vi "Teleop.vi"(10 "Match Info":T1={"Autonomous Elapsed Seconds"=0.0, "TeleOp Elapsed Seconds"=0.0, "Disabled Elapsed Seconds"=0.0, "Visited Autonomous"=FALSE, "Visited TeleOp"=FALSE, "Visited Disabled"=FALSE, "Autonomous Settings"={"Autonomous Style"=enum."Independent", "VI Refnum"=refnum}}, 11 "Call Context":T2) -> ()   [LabVIEW 2015]
doc: "This VI is called for each TeleOp packet received from the DS where the robot is not disabled. It is often used to read from the joysticks and update I/O or to update setpoints for timed control loops. It should complete and return within 20 milliseconds or it may miss DS packets."
uses:
  <vilib>/Rock Robotics/WPI/DriverStation/WPI_DriverStationDerivedRobotMode.ctl
  <vilib>/Rock Robotics/WPI/DriverStation/WPI_DriverStationMatch Info.ctl
  <vilib>/Rock Robotics/Network Tables/NT Read Boolean.vi
  <vilib>/Rock Robotics/Network Tables/NT Read Number.vi
  <vilib>/Rock Robotics/WPI/Utilities/WPI_GetSetVariantRefNum.vi
  Robot Global Data.vi
  <vilib>/Rock Robotics/Network Tables/NT Write Numeric Array.vi
  <vilib>/Rock Robotics/Network Tables/NT Write Boolean Array.vi
panel:
  in  "Fire":bool
  in  "Ball Intake":bool
  in  "Drive Mode":enum16{"Tank Drive", "Arcade Drive"}(ring)
  in  "Controller Mode":enum16{"X-Box Controller", "Joysticks"}(ring)
  out "Sample Slider 0":dbl(slide) scale=0.0..5.0
  out "Sample Boolean 1":bool
  out "Sample Boolean 0":bool
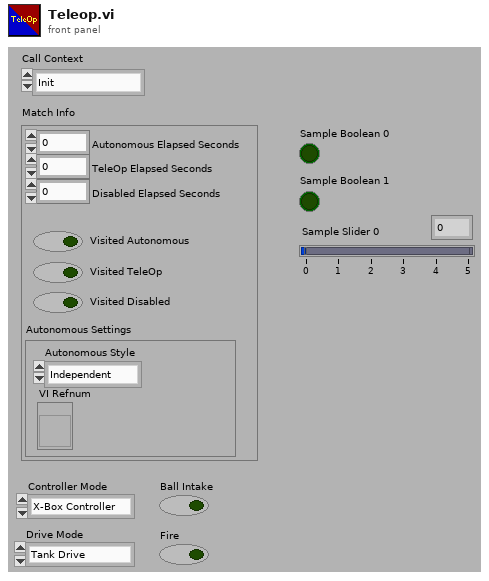
[diagram p1: front panel]
types:
  T1 = typedef "WPI_DriverStationMatch Info.ctl" = cluster{"Autonomous Elapsed Seconds":dbl, "TeleOp Elapsed Seconds":dbl, "Disabled Elapsed Seconds":dbl, "Visited Autonomous":bool, "Visited TeleOp":bool, "Visited Disabled":bool, "Autonomous Settings":cluster{"Autonomous Style":enum16{"Iterative", "Independent"}, "VI Refnum":refnum<vi>}}
  T2 = typedef "WPI_DriverStationDerivedRobotMode.ctl" = enum16{"Init", "Execute", "Stop"}
  T3 = typedef "WPI_RobotDriveDevRef.ctl" = cluster{"DevStatus":errorcluster, "Motors[]":T4[], "Square Inputs":bool, "Max Output":dbl}
  T4 = typedef "WPI_MotorControlDeviceRef.ctl" = cluster{"DeviceStatus":errorcluster, "Type":T5, "PWM":cluster{"PWM Channel":T6, "DeadBand":T7}, "CAN":cluster{"Device Number":u8, "Control Mode":T8, "Semaphore":T9, "Max Vout":dbl, "TalonSRX Control Mode":T10}, "Invert":bool}
  T5 = typedef "WPI_MotorControlType.ctl" = enum16{"PWM", "CAN", "CANTalonSRX"}
  T6 = typedef "FPGA_DIOPWMChannel.ctl" = enum8{"PWM 0", "PWM 1", "PWM 2", "PWM 3", "PWM 4", "PWM 5", "PWM 6", "PWM 7", "PWM 8", "PWM 9", "PWM MXP 0", "PWM MXP 1", "PWM MXP 2", "PWM MXP 3", "PWM MXP 4", "PWM MXP 5", "PWM MXP 6", "PWM MXP 7", "PWM MXP 8", "PWM MXP 9", "Invalid"}
  T7 = typedef "WPI_PWMDeadband.ctl" = cluster{"Name":string, "maxPositivePwm":i32, "minPositivePwm":i32, "centerPwm":i32, "maxNegativePwm":i32, "minNegativePwm":i32, "angularRange":u16}
  T8 = typedef "WPI_CANJaguar_ControlMode.ctl" = enum8{"Percent VBus", "Current", "Speed", "Position", "Voltage"}
  T9 = typedef "Semaphore RefNum" = refnum<k1>
  T10 = typedef "WPI_CANTalonSRX_APIControlMode.ctl" = enum8{"Percent VBus", "Speed", "Position", "Slave", "Unchanged / Invalid", "Voltage Compensation", "Current", "Motion Profile"}
  T11 = typedef "WPI_JoystickDevRef.ctl" = cluster{"Device":T12}
  T12 = typedef "WPI_JoystickDeviceEnum.ctl" = enum16{"USB 0", "USB 1", "USB 2", "USB 3", "USB 4", "USB 5"}
  T13 = cluster{"Ball Shooter Operation":enum16{"Ball Intake", "Fire Ball Shooter", "Aim Ball Shooter"}}
  T14 = enum16{"Ball Intake", "Fire Ball Shooter", "Aim Ball Shooter"}
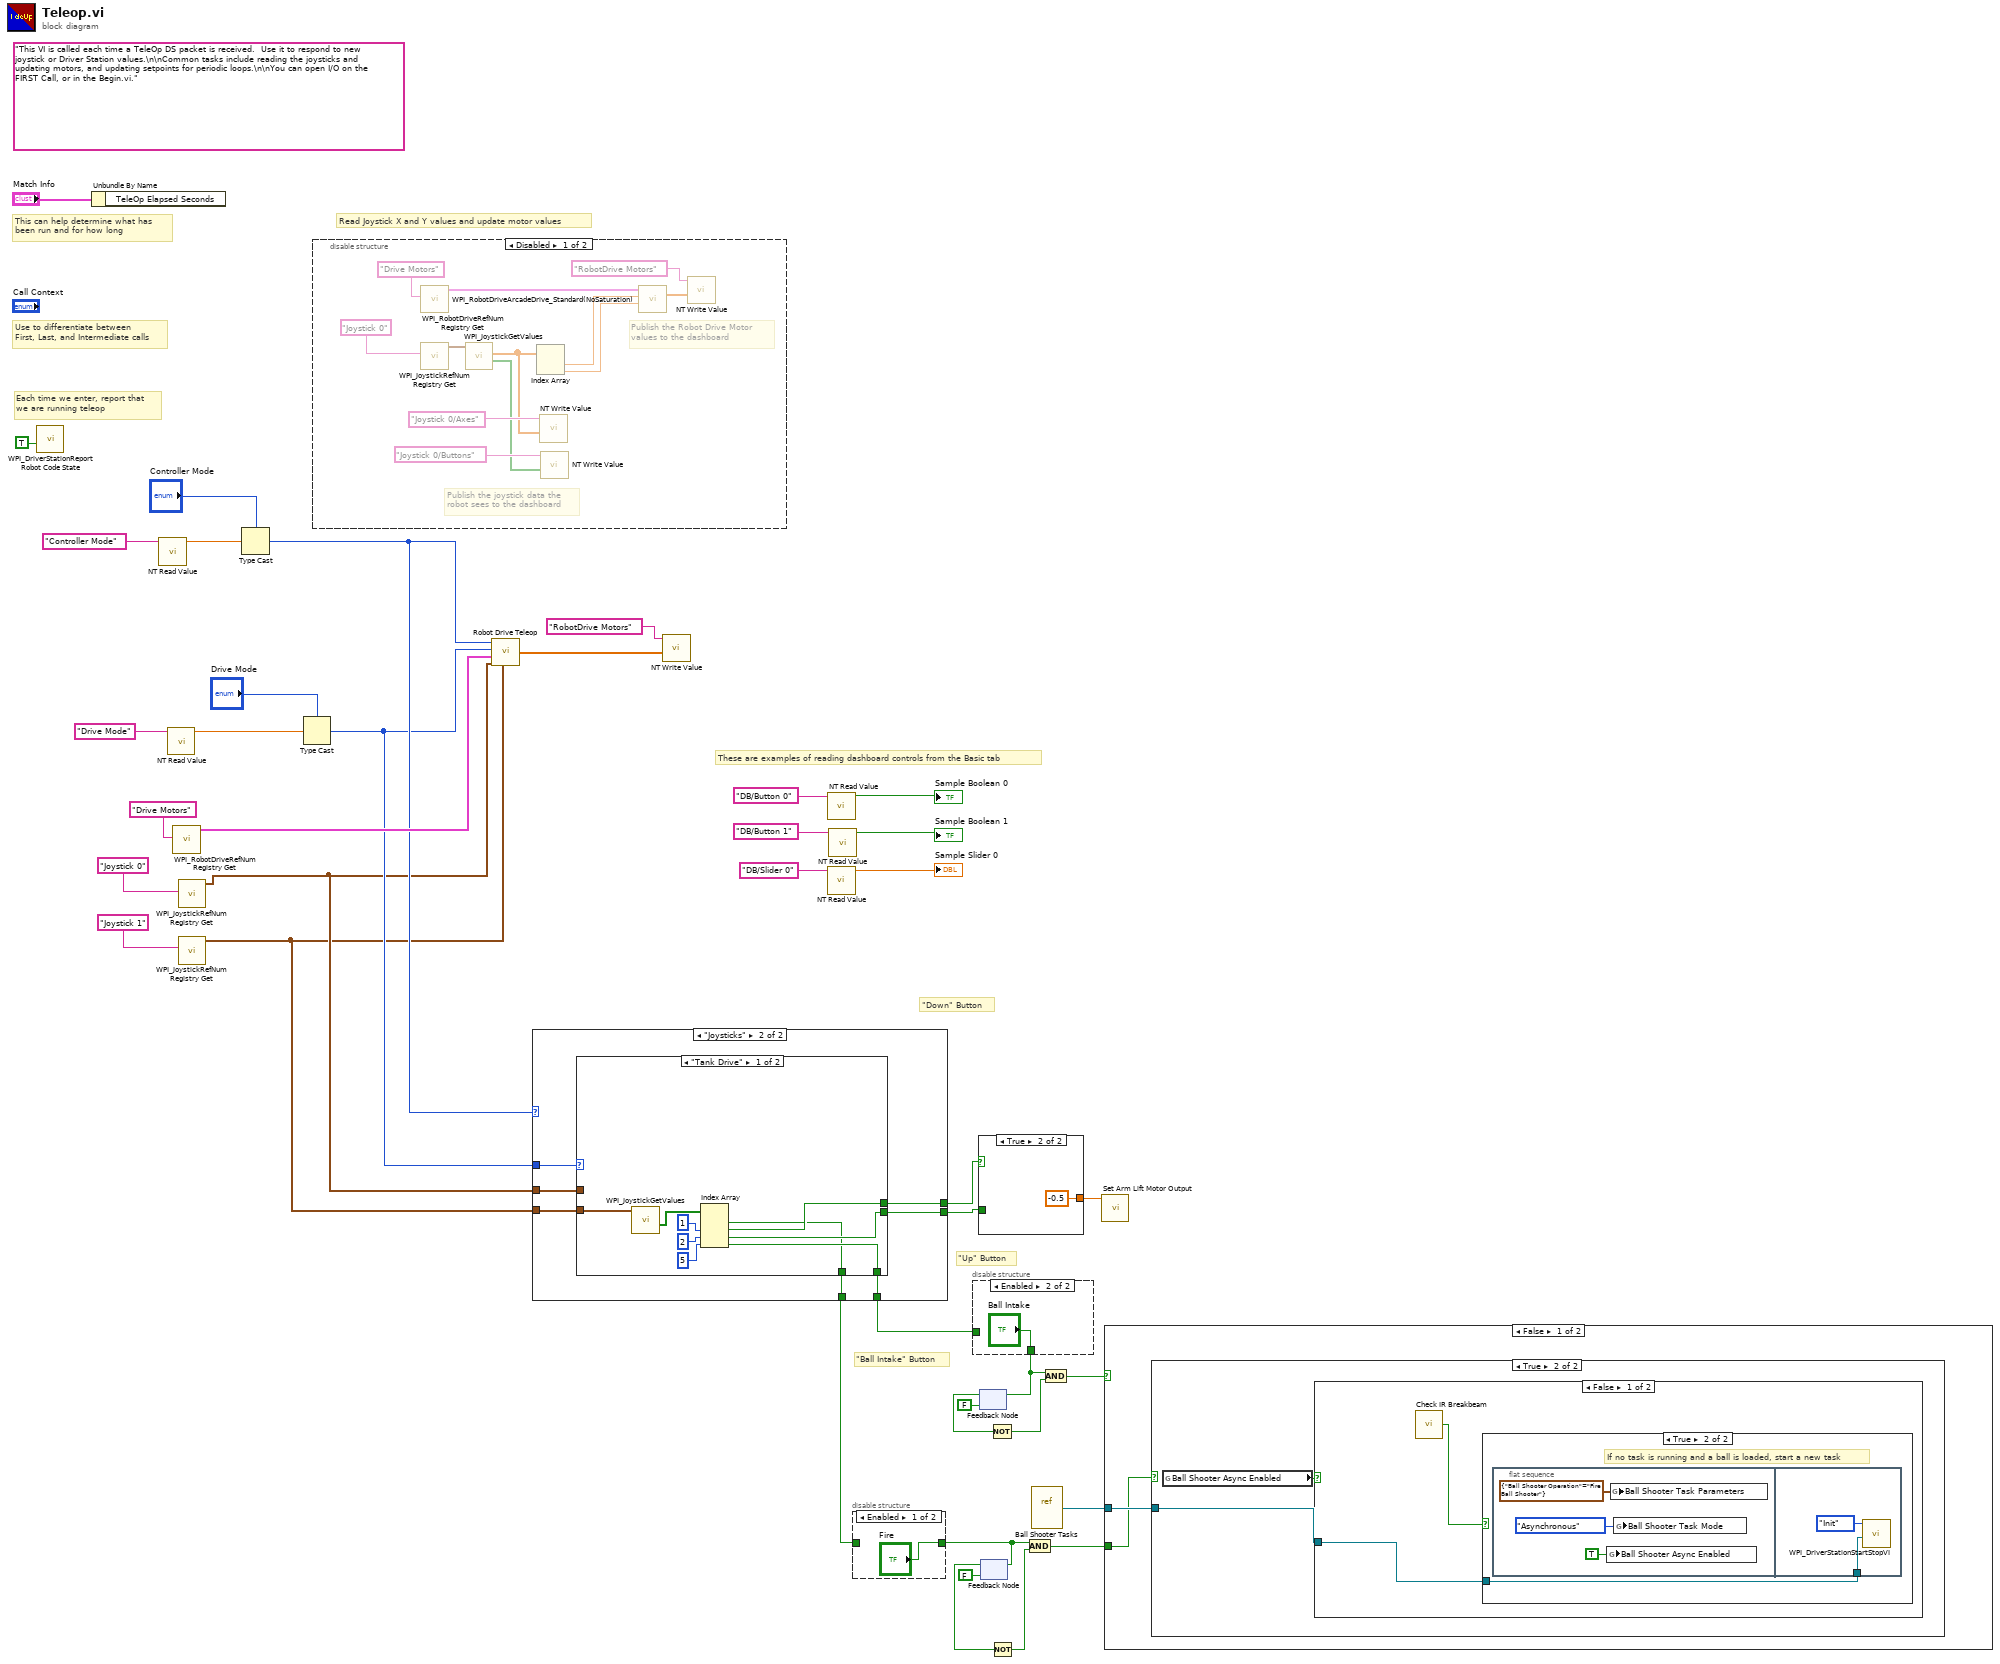
[diagram p0: block diagram]
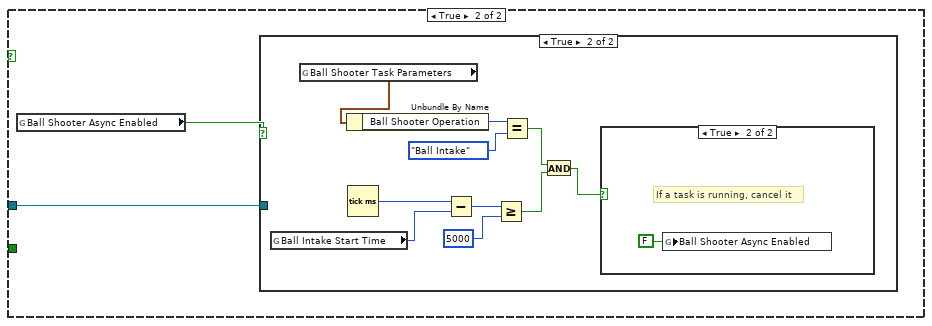
[diagram p7: hidden frame]
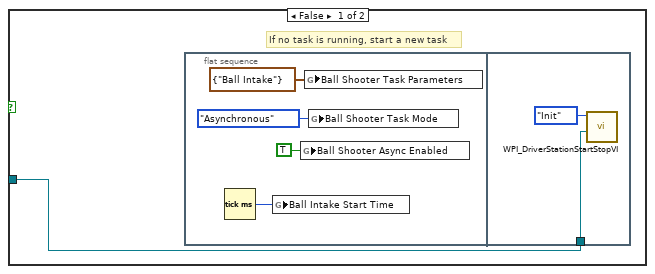
[diagram p8: hidden frame]
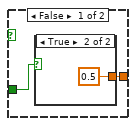
[diagram p10: hidden frame]
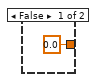
[diagram p11: hidden frame]
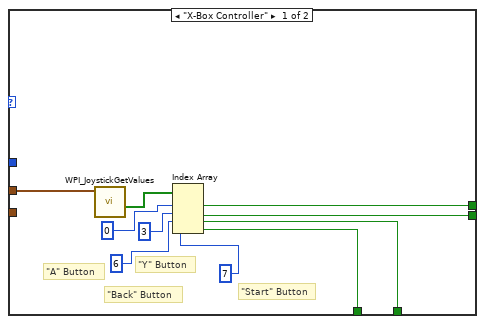
[diagram p12: hidden frame]
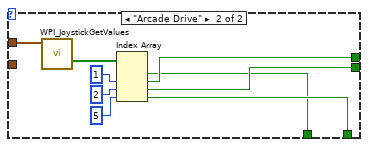
[diagram p13: hidden frame]
diagram:
  (unwired) "This VI is called each time a TeleOp DS packet is received.  Use it to respond to new joystick or Driver Station values.\n\nCommon tasks include reading the joysticks and updating motors, and updating setpoints for periodic loops.\n\nYou can open I/O on the FIRST Call, or in the Begin.vi."
  # "\"Ball Intake\" Button"
  # "\"Up\" Button"
  # "\"Down\" Button"
  # "These are examples of reading dashboard controls from the Basic tab"
  # "Each time we enter, report that\nwe are running teleop"
  # "Use to differentiate between\nFirst, Last, and Intermediate calls"
  # "This can help determine what has\nbeen run and for how long"
  # "Read Joystick X and Y values and update motor values"
  n1 = call <vilib>:"WPI_DriverStationReport Robot Code State.vi"("TeleOp"=TRUE ("Autonomous")) -> ()  [unwired: 10 in, 1 out]
  n2 = Unbundle By Name("Match Info") -> ()  [unwired: 1 out]
  n3 = call-poly <vilib>:"NT Read Value.vi"("Name"="Controller Mode") -> ("Numeric"=w31:dbl)  [unwired: 9 in, 1 out]
  n4 = call-poly <vilib>:"NT Read Value.vi"("Name"="Drive Mode") -> ("Numeric"=w27:dbl)  [unwired: 9 in, 1 out]
  n5 = call <vilib>:"WPI_RobotDriveRefNum Registry Get.vi"("refnum name"="Drive Motors") -> ("RobotDriveDevRef"=w25:T3)  [unwired: 1 in, 9 out]
  n6 = call <vilib>:"WPI_JoystickRefNum Registry Get.vi"("refnum name"="Joystick 0") -> ("JoystickDevRef"=w18:T11)  [unwired: 1 in, 9 out]
  n7 = call <vilib>:"WPI_JoystickRefNum Registry Get.vi"("refnum name"="Joystick 1") -> ("JoystickDevRef"=w17:T11)  [unwired: 1 in, 9 out]
  n8 = Type Cast(type="Controller Mode", x=w31) -> (*(type *) &x=w20:enum16{"X-Box Controller", "Joysticks"})
  n9 = Type Cast(type="Drive Mode", x=w27) -> (*(type *) &x=w19:enum16{"Tank Drive", "Arcade Drive"})
  n10 = disable-structure shown="Disabled" {
    frame Disabled {
      # "Publish the Robot Drive Motor\nvalues to the dashboard"
      # "Publish the joystick data the\nrobot sees to the dashboard"
      n11 = call <vilib>:"WPI_RobotDriveRefNum Registry Get.vi"("refnum name"="Drive Motors") -> ("RobotDriveDevRef"=w51:T3)  [unwired: 1 in, 9 out]
      n12 = call <vilib>:"WPI_JoystickRefNum Registry Get.vi"("refnum name"="Joystick 0") -> ("JoystickDevRef"=w48:T11)  [unwired: 1 in, 9 out]
      n13 = call <vilib>:"WPI_JoystickGetValues.vi"("JoystickDevRef"=w48) -> ("Buttons"=w43:bool[], "Axes"=w44:dbl[])  [unwired: 6 in, 3 out]
      n14 = Index Array(array=w44) -> (element #1=w50:dbl, element #2=w47:dbl)  [unwired: 2 in]
      n15 = call-poly <vilib>:"NT Write Value.vi"("Numeric Array"=w44, "Name"="Joystick 0/Axes") -> ()  [unwired: 9 in, 1 out]
      n16 = call-poly <vilib>:"NT Write Value.vi"("Boolean Array"=w43, "Name"="Joystick 0/Buttons") -> ()  [unwired: 9 in, 1 out]
      n17 = call <vilib>:"WPI_RobotDriveArcadeDrive_Standard(NoSaturation).vi"("Y axis value"=w47, "X axis value"=w50, "RobotDriveDevRef"=w51) -> ("Motor Values"=w42:dbl[])  [unwired: 1 in, 7 out]
      n18 = call-poly <vilib>:"NT Write Value.vi"("Numeric Array"=w42, "Name"="RobotDrive Motors") -> ()  [unwired: 9 in, 1 out]
    }
    frame Enabled {
    }
  }
  n19 = call "Robot Drive Teleop.vi"("Controller Mode"=w20, "Drive Mode"=w19, "RobotDriveDevRef"=w25, "Joystick0DevRef"=w18, "Joystick1DevRef"=w17) -> ("Motor Values"=w21:dbl[])
  n20 = case shown="\"Joysticks\"" w20 {
    tunnel: w19 -> [_ w69]
    tunnel: w18 -> [w62 w68]
    tunnel: w17 -> [_ w65]
    tunnel: [w58 w67] -> w16
    tunnel: [w57 w66] -> w15
    tunnel: [w55 w64] -> w7
    tunnel: [w54 w63] -> w1
    frame "X-Box Controller" {
      # "\"Start\" Button"
      # "\"Back\" Button"
      # "\"Y\" Button"
      # "\"A\" Button"
      n21 = call <vilib>:"WPI_JoystickGetValues.vi"("JoystickDevRef"=w62) -> ("Buttons"=w61:bool[])  [unwired: 6 in, 4 out]
      n22 = Index Array(array=w61, index #1=0 ("index"), index #2=3 ("index"), index #3=6 ("index"), index #4=7 ("index")) -> (element #1=w58:bool, element #2=w57:bool, element #3=w55:bool, element #4=w54:bool)
    }
    frame "Joysticks" {
      n23 = case shown="\"Tank Drive\"" w69 {
        tunnel: w68 -> [_ w87]
        tunnel: [w71 w80] -> w67
        tunnel: [w72 w81] -> w66
        tunnel: w65 -> [w77 _]
        tunnel: [w73 w82] -> w64
        tunnel: [w70 w79] -> w63
        frame "Tank Drive" {
          n24 = call <vilib>:"WPI_JoystickGetValues.vi"("JoystickDevRef"=w77) -> ("Buttons"=w78:bool[])  [unwired: 6 in, 4 out]
          n25 = Index Array(array=w78, index #2=1 ("index"), index #3=2 ("index"), index #4=5 ("index")) -> (element #1=w70:bool, element #2=w71:bool, element #3=w72:bool, element #4=w73:bool)  [unwired: 1 in]
        }
        frame "Arcade Drive" {
          n26 = call <vilib>:"WPI_JoystickGetValues.vi"("JoystickDevRef"=w87) -> ("Buttons"=w83:bool[])  [unwired: 6 in, 4 out]
          n27 = Index Array(array=w83, index #2=1 ("index"), index #3=2 ("index"), index #4=5 ("index")) -> (element #1=w79:bool, element #2=w80:bool, element #3=w81:bool, element #4=w82:bool)  [unwired: 1 in]
        }
      }
    }
  }
  n28 = call-poly <vilib>:"NT Write Value.vi"("Numeric Array"=w21, "Name"="RobotDrive Motors") -> ()  [unwired: 9 in, 1 out]
  n29 = call-poly <vilib>:"NT Read Value.vi"("Name"="DB/Button 0" ("refnum name")) -> ("Boolean"=→"Sample Boolean 0":bool)  [unwired: 9 in, 1 out]
  n30 = call-poly <vilib>:"NT Read Value.vi"("Name"="DB/Slider 0" ("refnum name")) -> ("Numeric"=→"Sample Slider 0":dbl)  [unwired: 9 in, 1 out]
  n31 = call-poly <vilib>:"NT Read Value.vi"("Name"="DB/Button 1" ("refnum name")) -> ("Boolean"=→"Sample Boolean 1":bool)  [unwired: 9 in, 1 out]
  n32 = disable-structure shown="Enabled" {
    disable-tunnel: ["Fire" w89] -> w2
    disable-tunnel: w1 -> [_ w89]
    frame Enabled {
    }
    frame Disabled {
    }
  }
  n33 = disable-structure shown="Enabled" {
    disable-tunnel: [w90 "Ball Intake"] -> w8
    disable-tunnel: w7 -> [w90 _]
    frame Disabled {
    }
    frame Enabled {
    }
  }
  n34 = case shown="True" w16 {
    tunnel: w15 -> [w93 _]
    tunnel: [w92 -0.5] -> w14
    frame False {
      n35 = case shown="True" w93 {
        tunnel: [0.0 0.5] -> w92
        frame False {
        }
        frame True {
        }
      }
    }
    frame True {
    }
  }
  n36 = feedback-in #1(w8) -> ()
  n37 = feedback #1(FALSE) -> (w12:bool)
  n38 = feedback #2(FALSE) -> (w5:bool)
  n39 = feedback-in #2(w2) -> ()
  n40 = Not(x=w12) -> (.not. x?=w11:bool)
  n41 = Not(x=w5) -> (.not. x?=w6:bool)
  n42 = And(x=w2, y=w6) -> (x .and. y?=w3:bool)
  n43 = vi-ref "Ball Shooter Tasks.vi"() -> (w9:refnum<vi>)
  n44 = And(x=w8, y=w11) -> (x .and. y?=w10:bool)
  n45 = call "Set Arm Lift Motor Output.vi"("Output"=w14) -> ()  [unwired: 3 out]
  n46 = case shown="False" w10 {
    tunnel: w9 -> [w98 w109]
    tunnel: w3 -> [w97 _]
    frame False {
      n47 = case shown="True" w97 {
        tunnel: w98 -> [_ w99]
        frame False {
        }
        frame True {
          n48 = global read "Robot Global Data.vi" "Ball Shooter Async Enabled"() -> (w100:bool)
          n49 = case shown="False" w100 {
            tunnel: w99 -> [w102 _]
            frame False {
              n50 = call "Check IR Breakbeam.vi"() -> ("Beam Broken"=w101:bool)
              n51 = case shown="True" w101 {
                tunnel: w102 -> [_ w103]
                frame False {
                }
                frame True {
                  # "If no task is running and a ball is loaded, start a new task"
                  n52 = flat-sequence {
                    tunnel: w103 -> [w107]
                    frame #0 {
                      n53 = global write "Robot Global Data.vi" "Ball Shooter Async Enabled"(TRUE ("Ball Shooter Async Enabled")) -> ()
                      n54 = global write "Robot Global Data.vi" "Ball Shooter Task Parameters"(T13 {"Ball Shooter Operation"=enum."Fire Ball Shooter"} ("Ball Shooter Task Parameters")) -> ()
                      n55 = global write "Robot Global Data.vi" "Ball Shooter Task Mode"(enum16{"Synchronous", "Asynchronous"}."Asynchronous" ("Ball Shooter Task Mode")) -> ()
                    }
                    frame #1 {
                      n56 = call <vilib>:"WPI_DriverStationStartStopVI.vi"("VI in"=w107, "Call Context"=WPI_DriverStationDerivedRobotMode."Init") -> ()  [unwired: 10 in]
                    }
                  }
                }
              }
            }
            frame True {
              # "Ignore the button press if the ball shooter is already running"
            }
          }
        }
      }
    }
    frame True {
      n57 = global read "Robot Global Data.vi" "Ball Shooter Async Enabled"() -> (w110:bool)
      n58 = case shown="True" w110 {
        tunnel: w109 -> [w111 _]
        frame False {
          # "If no task is running, start a new task"
          n59 = flat-sequence {
            tunnel: w111 -> [w116]
            frame #0 {
              n60 = Tick Count (ms)() -> (millisecond timer value=w112:u32)
              n61 = global write "Robot Global Data.vi" "Ball Intake Start Time"(w112) -> ()
              n62 = global write "Robot Global Data.vi" "Ball Shooter Async Enabled"(TRUE ("Ball Shooter Async Enabled")) -> ()
              n63 = global write "Robot Global Data.vi" "Ball Shooter Task Parameters"(T13 {"Ball Shooter Operation"=enum."Ball Intake"} ("Ball Shooter Task Parameters")) -> ()
              n64 = global write "Robot Global Data.vi" "Ball Shooter Task Mode"(enum16{"Synchronous", "Asynchronous"}."Asynchronous" ("Ball Shooter Task Mode")) -> ()
            }
            frame #1 {
              n65 = call <vilib>:"WPI_DriverStationStartStopVI.vi"("VI in"=w116, "Call Context"=WPI_DriverStationDerivedRobotMode."Init") -> ()  [unwired: 10 in]
            }
          }
        }
        frame True {
          n66 = global read "Robot Global Data.vi" "Ball Intake Start Time"() -> (w123:u32)
          n67 = global read "Robot Global Data.vi" "Ball Shooter Task Parameters"() -> (w127:T13)
          n68 = Unbundle By Name(w127) -> ("Ball Shooter Operation"=w126:T14)
          n69 = Tick Count (ms)() -> (millisecond timer value=w124:u32)
          n70 = Subtract(x=w124, y=w123) -> (x-y=w122:u32)
          n71 = Greater Or Equal?(x=w122, y=u32 5000) -> (x >= y?=w119:bool)
          n72 = Equal?(x=w126, y=T14."Ball Intake") -> (x = y?=w120:bool)
          n73 = And(x=w120, y=w119) -> (x .and. y?=w118:bool)
          n74 = case shown="True" w118 {
            frame False {
            }
            frame True {
              # "If a task is running, cancel it"
              n75 = global write "Robot Global Data.vi" "Ball Shooter Async Enabled"(FALSE ("Ball Shooter Async Enabled")) -> ()
            }
          }
        }
      }
    }
  }
